vi "PathToINIFiles.vi"(7 "Boolean":bool, 11 "IniFilePaths In":path[](array[path])) -> (3 "IniFilePaths Out":path[](array[path]))   [LabVIEW 2018]
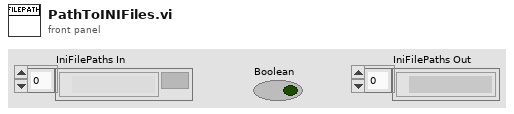
[diagram p1: front panel]
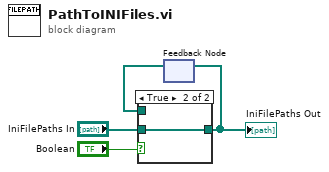
[diagram p0: block diagram]
diagram:
  n1 = feedback #1() -> (w4:path[])  [unwired: 1 in]
  n2 = case shown="True" "Boolean" {
    tunnel: "IniFilePaths In" -> [_ w6]
    tunnel: [w5 w6] -> w1
    tunnel: w4 -> [w5 _]
    frame False {
    }
    frame True {
    }
  }
  "IniFilePaths Out" <- w1
  n3 = feedback-in #1(w1) -> ()
